vi "Probe (Cluster).vi"(9 "Data Valid":bool, 10 "Acquisition Status":T1={"Reset"=FALSE, "Acquisition Engine Start (Arm)"=FALSE, "Current State"=enum."Acquire Pre-Trigger Samples", "Trig Offset"=0, "Points Unread"=0, "Points Acquired"=0, "Records Done"=0, "Start of Read"=FALSE, "End of Read"=FALSE, "Start of Record"=FALSE, "End of Record"=FALSE, "Ready for Ref Trig"=FALSE, "In Reset?"=FALSE}) -> (1 "Address":u64, 2 "Collected Data":T1[](array[typedef]))   [LabVIEW 2011]
uses:
  <userlib>/OCT Reference Design/Acquisition Engine/Acquisition Status.ctl
  <userlib>/OCT Reference Design/Acquisition Engine/Acquisition Engine State.ctl
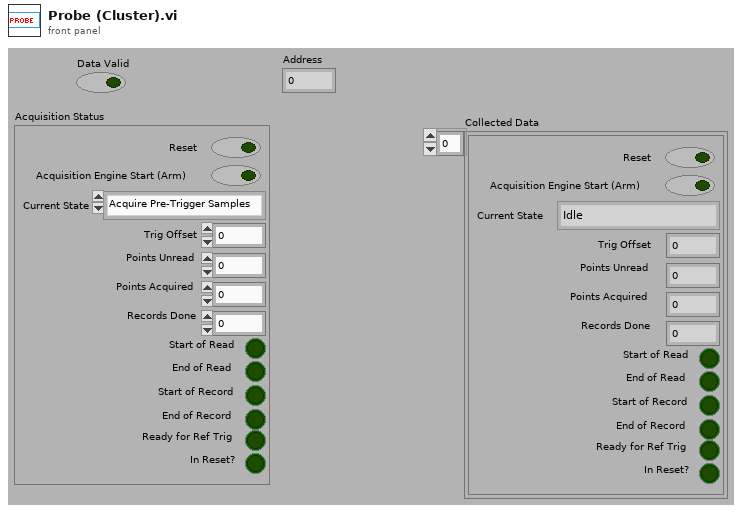
[diagram p1: front panel]
types:
  T1 = typedef "Acquisition Status.ctl" = cluster{"Reset":bool, "Acquisition Engine Start (Arm)":bool, "Current State":T2, "Trig Offset":u8, "Points Unread":u16, "Points Acquired":u16, "Records Done":u16, "Start of Read":bool, "End of Read":bool, "Start of Record":bool, "End of Record":bool, "Ready for Ref Trig":bool, "In Reset?":bool}
  T2 = typedef "Acquisition Engine State.ctl" = enum16{"Idle", "Arm Acquisition Engine", "Acquire Pre-Trigger Samples", "Wait for Trigger", "Acquisition Hold Off Time", "Read Data from Buffer", "Check Records Done?", "Re-Arm State", "Flush Available Data"}
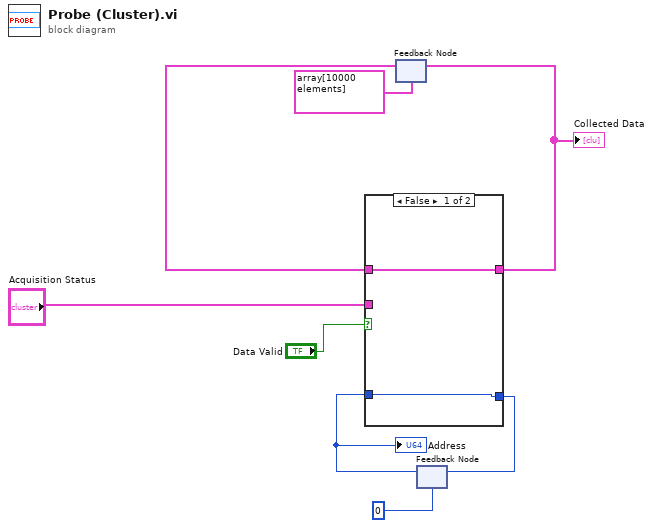
[diagram p0: block diagram]
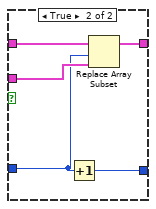
[diagram p2: hidden frame]
diagram:
  n1 = feedback #1(T1[] array[10000 elements]) -> (w8:T1[])
  n2 = feedback #2(u64 0) -> (w2:u64)
  "Address" <- w2
  n3 = case shown="False" "Data Valid" {
    tunnel: "Acquisition Status" -> [_ w15]
    tunnel: w8 -> [w10 w14]
    tunnel: [w10 w13] -> w7
    tunnel: w2 -> [w9 w11]
    tunnel: [w9 w12] -> w4
    frame False {
    }
    frame True {
      n4 = Increment(x=w11) -> (x+1=w12:u64)
      n5 = Replace Array Subset(array=w14, new element=w15, index=w11) -> (w13:T1[])
    }
  }
  "Collected Data" <- w7
  n6 = feedback-in #1(w7) -> ()
  n7 = feedback-in #2(w4) -> ()
